vi "Format JSON String.vi"(11 "Key in":string) -> (3 "Key out":string)   [LabVIEW 2020]
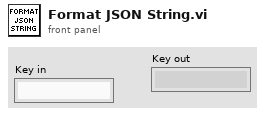
[diagram p1: front panel]
types:
  T1 = cluster{"replace string (\"\")":string, "replace string (\"\") 2":string}[]
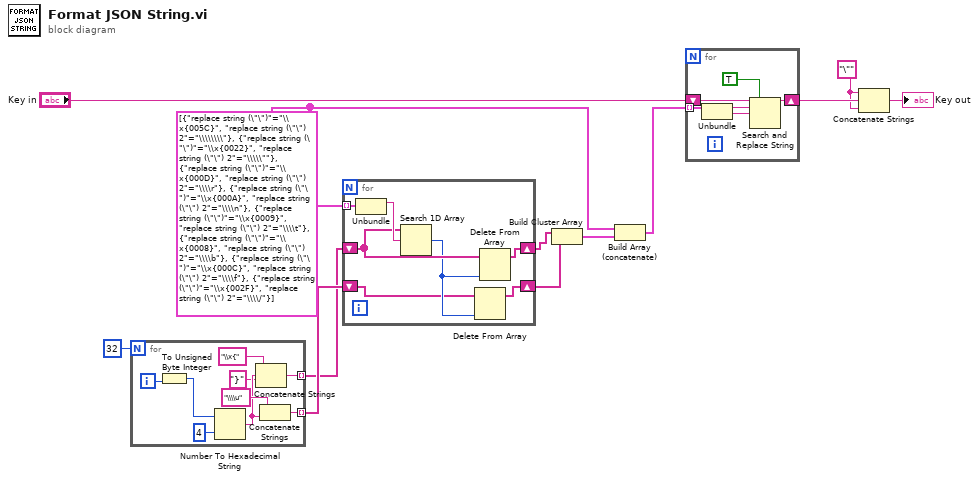
[diagram p0: block diagram]
diagram:
  w11 = "\"" ("string")
  w7 = T1 [{"replace string (\"\")"="\\x{005C}", "replace string (\"\") 2"="\\\\\\\\"}, {"replace string (\"\")"="\\x{0022}", "replace string (\"\") 2"="\\\\\""}, {"replace string (\"\")"="\\x{000D}", "replace string (\"\") 2"="\\\\r"}, {"replace string (\"\")"="\\x{000A}", "replace string (\"\") 2"="\\\\n"}, {"replace string (\"\")"="\\x{0009}", "replace string (\"\") 2"="\\\\t"}, {"replace string (\"\")"="\\x{0008}", "replace string (\"\") 2"="\\\\b"}, {"replace string (\"\")"="\\x{000C}", "replace string (\"\") 2"="\\\\f"}, {"replace string (\"\")"="\\x{002F}", "replace string (\"\") 2"="\\\\/"}]
  n1 = for {
    N: 32 -> [_]
    tunnel: [w18] -> w3 mode=indexing
    tunnel: [w13] -> w2 mode=indexing
    i -> [w21]
    n2 = To Unsigned Byte Integer(number=w21) -> (unsigned 8bit integer=w16:u8)
    n3 = Number To Hexadecimal String(1:i16 4 ("width (-)"), 2:w16) -> (0:w15:string)
    n4 = Concatenate Strings("\\x{" ("string"), w15, "}" ("string")) -> (w13:string)
    n5 = Concatenate Strings("\\\\u" ("string"), w15) -> (w18:string)
  }
  n6 = for {
    tunnel: w7 -> [w28] mode=indexing
    shift-right: [w26] -> w5
    shift-left: w2 -> [w25]
    shift-right: [w23] -> w1
    shift-left: w3 -> [w22]
    n7 = Unbundle(w28) -> ("replace string (\"\")"=w27:string)  [unwired: 1 out]
    n8 = Search 1D Array(1D array=w25, element=w27) -> (index of element=w24:i32)  [unwired: 1 in]
    n9 = Delete From Array(array=w22, index=w24) -> (array with subset deleted=w23:string[])  [unwired: 1 in, 1 out]
    n10 = Delete From Array(array=w25, index=w24) -> (array with subset deleted=w26:string[])  [unwired: 1 in, 1 out]
  }
  n11 = Build Cluster Array(w5, w1) -> (w8:cluster{string, string}[])
  n12 = Build Array (concatenate)(w7, w8) -> (w6:T1)
  n13 = for {
    tunnel: w6 -> [w32] mode=indexing
    shift-right: [w29] -> w12
    shift-left: "Key in" -> [w34]
    n14 = Unbundle(w32) -> ("replace string (\"\")"=w31:string, "replace string (\"\") 2"=w30:string)
    n15 = Search and Replace String(replace all?=TRUE ("replace all? (F)"), input string=w34, search string=w31, replace string=w30) -> (result string=w29:string)  [unwired: 4 in, 3 out]
  }
  n16 = Concatenate Strings(w11, w12, w11) -> (→"Key out":string)
